vi "VariablesTCMouseDown.vi"(8 "error in (no error)":errorcluster, 10 "MouseDownIn":T3, 11 "VMUI in":refnum<class "VMUI.lvclass">) -> (0 "error out":errorcluster, 2 "MouseDownOut":T1, 3 "VMUI out":refnum<class "VMUI.lvclass">)   [LabVIEW 2013, in "VMUI.lvclass"]
uses:
  VMUI.lvclass
  <vilib>/Utility/miscctls.llb/LVPoint32TypeDef.ctl
  <vilib>/Utility/miscctls.llb/LVRowAndColumnTypeDef.ctl
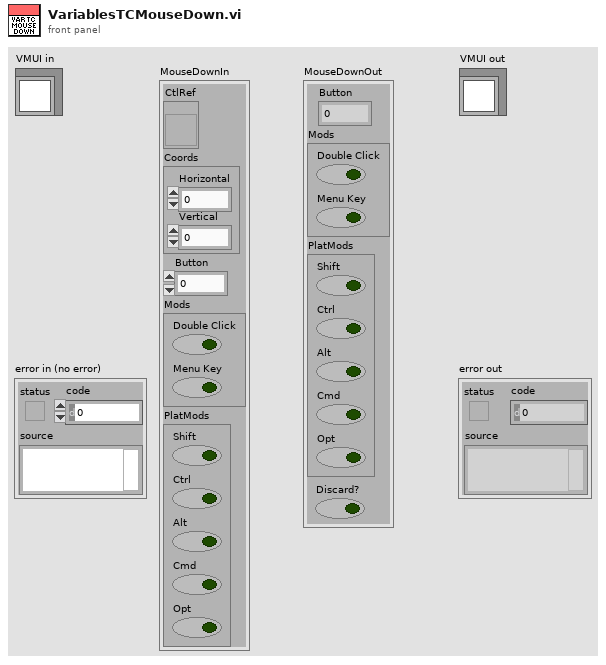
[diagram p1: front panel]
types:
  T1 = cluster{"Button":u16, "Mods":cluster{"Double Click":bool, "Menu Key":bool}, "PlatMods":cluster{"Shift":bool, "Ctrl":bool, "Alt":bool, "Cmd":bool, "Opt":bool}, "Discard?":bool}
  T2 = typedef "LVPoint32TypeDef.ctl" = cluster{"Horizontal":i32, "Vertical":i32}
  T3 = cluster{"CtlRef":refnum<vi>, "Coords":T2, "Button":u16, "Mods":cluster{"Double Click":bool, "Menu Key":bool}, "PlatMods":cluster{"Shift":bool, "Ctrl":bool, "Alt":bool, "Cmd":bool, "Opt":bool}}
  T4 = typedef "LVRowAndColumnTypeDef.ctl" = cluster{"Row":i32, "Column":i32}
  T5 = cluster{"Shift":bool, "Ctrl":bool, "Alt":bool, "Cmd":bool, "Opt":bool}
  T6 = cluster{"Button":u16, "Mods":cluster{"Double Click":bool, "Menu Key":bool}, "PlatMods":cluster{"Shift":bool, "Ctrl":bool, "Alt":bool, "Cmd":bool, "Opt":bool}, bool}
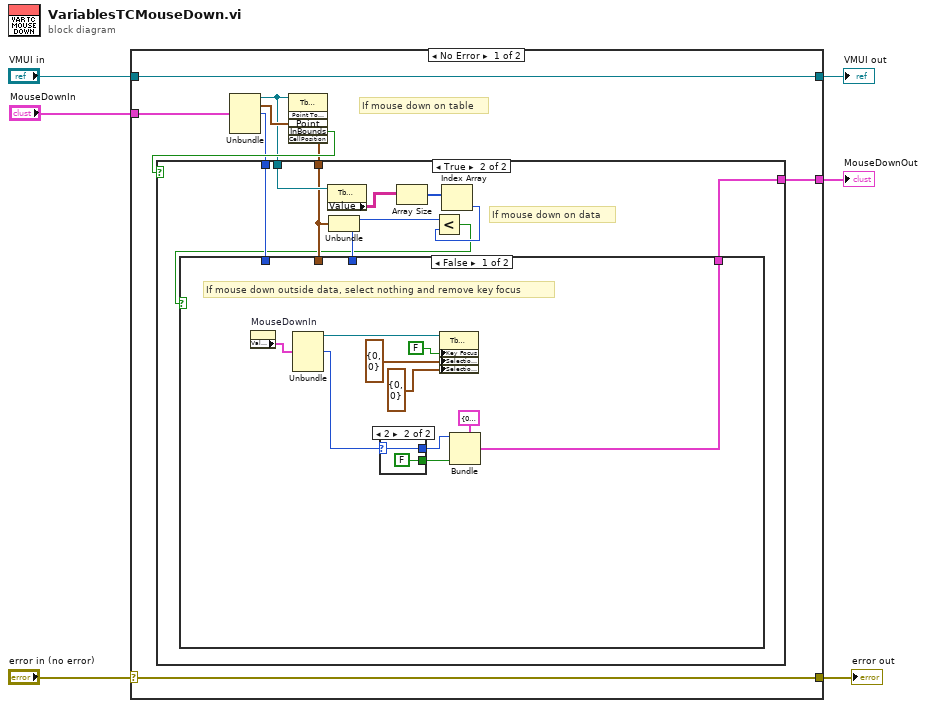
[diagram p0: block diagram]
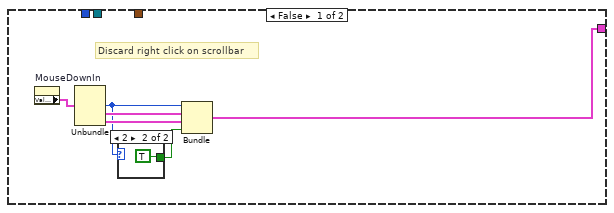
[diagram p2: hidden frame]
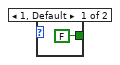
[diagram p3: hidden frame]
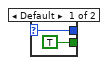
[diagram p4: hidden frame]
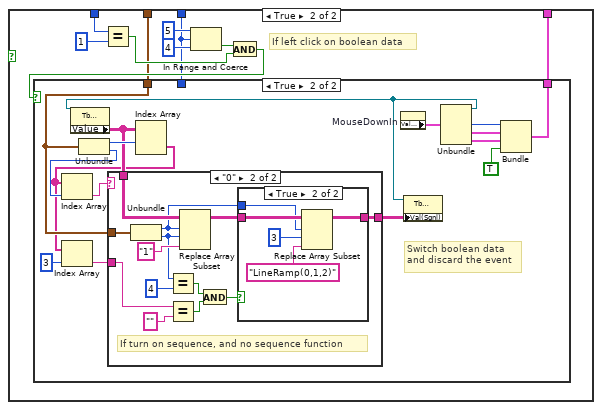
[diagram p5: hidden frame]
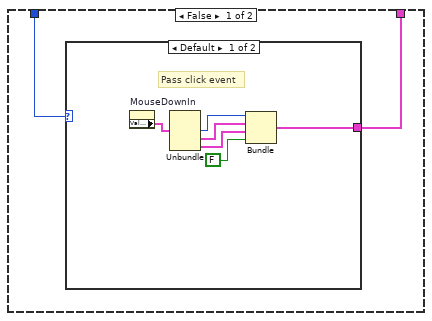
[diagram p6: hidden frame]
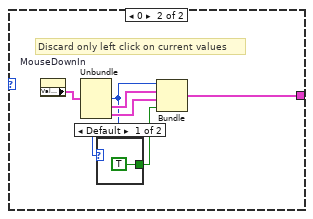
[diagram p7: hidden frame]
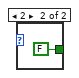
[diagram p8: hidden frame]
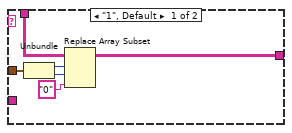
[diagram p9: hidden frame]
diagram:
  n1 = case shown="No Error" "error in (no error)" {
    selector: "error in (no error)" -> [w14 w116]
    tunnel: [w14 w116] -> w5
    tunnel: [w15 w115] -> w1
    tunnel: "VMUI in" -> [w15 w115]
    tunnel: "MouseDownIn" -> [w8 _]
    tunnel: [w7 _] -> w3
    frame No Error {
      # "If mouse down on table"
      n2 = Unbundle(w8) -> ("CtlRef"=w9:refnum<vi>, "Coords"=w13:T2, "Button"=w10:u16)  [unwired: 2 out]
      n3 = invoke class="Tbl (strict)" method="Point To Row Column"(reference=w9, "Point"=w13) -> ("InBounds"=w12:bool, "CellPosition"=w11:T4)  [unwired: 4 in, 4 out]
      n4 = case shown="True" w12 {
        tunnel: [w21 w29] -> w7
        tunnel: w11 -> [_ w26]
        tunnel: w9 -> [_ w28]
        tunnel: w10 -> [_ w27]
        frame False {
          # "Discard right click on scrollbar"
          n5 = property on="MouseDownIn" class="Clust (strict)"() -> ("Value"=w20:T3)  [unwired: 2 in, 2 out]
          n6 = Unbundle(w20) -> ("Button"=w17:u16, "Mods"=w19:cluster{"Double Click":bool, "Menu Key":bool}, "PlatMods"=w18:T5)  [unwired: 2 out]
          n7 = case shown="2" w17 {
            tunnel: [FALSE TRUE] -> w16
            frame 1, Default {
            }
            frame 2 {
            }
          }
          n8 = Bundle("Button"=w17, "Mods"=w19, "PlatMods"=w18, w16) -> (w21:T6)  [unwired: 1 in]
        }
        frame True {
          # "If mouse down on data"
          n9 = property class="Tbl (strict)"(reference=w28) -> ("Value"=w33:string[][])  [unwired: 1 in, 2 out]
          n10 = Unbundle(w26) -> ("Row"=w30:i32, "Column"=w25:i32)
          n11 = Array Size(array=w33) -> (size(s)=w32:i32[])
          n12 = Index Array(array=w32) -> (element=w31:i32)  [unwired: 1 in]
          n13 = Less?(x=w30, y=w31) -> (x < y?=w24:bool)
          n14 = case shown="False" w24 {
            tunnel: [w42 w55] -> w29
            tunnel: w25 -> [_ w48]
            tunnel: w27 -> [_ w54]
            tunnel: w26 -> [_ w49]
            frame False {
              # "If mouse down outside data, select nothing and remove key focus"
              n15 = property on="MouseDownIn" class="Clust (strict)"() -> ("Value"=w43:T3)  [unwired: 2 in, 2 out]
              n16 = Unbundle(w43) -> ("CtlRef"=w41:refnum<vi>, "Button"=w37:u16)  [unwired: 3 out]
              n17 = case shown="2" w37 {
                selector: w37 -> [w45 w46]
                tunnel: [TRUE FALSE] -> w36
                tunnel: [w45 w46] -> w35
                frame Default {
                }
                frame 2 {
                }
              }
              n18 = property class="Tbl (strict)"(reference=w41, "Key Focus"=FALSE, "Selection Size"=T4 {"Row"=0, "Column"=0}, "Selection Start"=T4 {"Row"=0, "Column"=0}) -> ()  [unwired: 1 in, 2 out]
              n19 = Bundle(cluster=T1 {"Button"=0, "Mods"={"Double Click"=FALSE, "Menu Key"=FALSE}, "PlatMods"={"Shift"=FALSE, "Ctrl"=FALSE, "Alt"=FALSE, "Cmd"=FALSE, "Opt"=FALSE}, "Discard?"=TRUE} ("MouseDownOut"), "Button"=w35, "Discard?"=w36) -> (w42:T1)  [unwired: 2 in]
            }
            frame True {
              # "If left click on boolean data"
              n20 = Equal?(x=w54, y=u16 1) -> (x = y?=w50:bool)
              n21 = In Range and Coerce(upper limit=5, x=w48, lower limit=4 ("upper limit")) -> (In Range?=w52:bool)  [unwired: 1 out]
              n22 = And(x=w52, y=w50) -> (x .and. y?=w51:bool)
              n23 = case shown="True" w51 {
                tunnel: [w59 w84] -> w55
                tunnel: w49 -> [_ w81]
                tunnel: w48 -> [w58 _]
                frame False {
                  n24 = case shown="Default" w58 {
                    tunnel: [w62 w67] -> w59
                    frame Default {
                      # "Pass click event"
                      n25 = property on="MouseDownIn" class="Clust (strict)"() -> ("Value"=w65:T3)  [unwired: 2 in, 2 out]
                      n26 = Unbundle(w65) -> ("Button"=w61:u16, "Mods"=w64:cluster{"Double Click":bool, "Menu Key":bool}, "PlatMods"=w63:T5)  [unwired: 2 out]
                      n27 = Bundle("Button"=w61, "Mods"=w64, "PlatMods"=w63, FALSE) -> (w62:T6)  [unwired: 1 in]
                    }
                    frame 0 {
                      # "Discard only left click on current values"
                      n28 = property on="MouseDownIn" class="Clust (strict)"() -> ("Value"=w70:T3)  [unwired: 2 in, 2 out]
                      n29 = Unbundle(w70) -> ("Button"=w66:u16, "Mods"=w69:cluster{"Double Click":bool, "Menu Key":bool}, "PlatMods"=w68:T5)  [unwired: 2 out]
                      n30 = case shown="Default" w66 {
                        tunnel: [TRUE FALSE] -> w71
                        frame Default {
                        }
                        frame 2 {
                        }
                      }
                      n31 = Bundle("Button"=w66, "Mods"=w69, "PlatMods"=w68, w71) -> (w67:T6)  [unwired: 1 in]
                    }
                  }
                }
                frame True {
                  # "Switch boolean data \nand discard the event"
                  n32 = Unbundle(w81) -> ("Row"=w83:i32, "Column"=w79:i32)
                  n33 = property on="MouseDownIn" class="Clust (strict)"() -> ("Value"=w88:T3)  [unwired: 2 in, 2 out]
                  n34 = Unbundle(w88) -> ("CtlRef"=w74:refnum<vi>, "Button"=w87:u16, "Mods"=w86:cluster{"Double Click":bool, "Menu Key":bool}, "PlatMods"=w85:T5)  [unwired: 1 out]
                  n35 = property class="Tbl (strict)"(reference=w74) -> ("Value"=w82:string[][])  [unwired: 1 in, 2 out]
                  n36 = Index Array(array=w82, index (row)=w83) -> (element=w77:string[])  [unwired: 1 in]
                  n37 = Index Array(array=w77, index=w79) -> (element=w78:string)
                  n38 = Index Array(array=w77, index=3) -> (element=w75:string)
                  n39 = case shown="\"0\"" w78 {
                    tunnel: w82 -> [w95 w104]
                    tunnel: w81 -> [w94 w108]
                    tunnel: [w90 w98] -> w80
                    tunnel: w75 -> [_ w103]
                    frame "1", Default {
                      n40 = Unbundle(w94) -> ("Row"=w93:i32, "Column"=w92:i32)
                      n41 = Replace Array Subset(array=w95, new element="0" ("new element/subarray"), index (row)=w93, index (col)=w92) -> (w90:string[][])
                    }
                    frame "0" {
                      # "If turn on sequence, and no sequence function"
                      n42 = Unbundle(w108) -> ("Row"=w96:i32, "Column"=w106:i32)
                      n43 = Equal?(x=w106, y=4) -> (x = y?=w101:bool)
                      n44 = Equal?(x=w103, y="") -> (x = y?=w100:bool)
                      n45 = Replace Array Subset(array=w104, new element="1" ("new element/subarray"), index (row)=w96, index (col)=w106) -> (w99:string[][])
                      n46 = And(x=w101, y=w100) -> (x .and. y?=w97:bool)
                      n47 = case shown="True" w97 {
                        tunnel: w99 -> [w109 w114]
                        tunnel: [w109 w113] -> w98
                        tunnel: w96 -> [_ w112]
                        frame False {
                        }
                        frame True {
                          n48 = Replace Array Subset(array=w114, new element="LineRamp(0,1,2)", index (row)=w112, index (col)=3 ("disabled index (col)")) -> (w113:string[][])
                        }
                      }
                    }
                  }
                  n49 = property class="Tbl (strict)"(reference=w74, "Val(Sgnl)"=w80) -> ()  [unwired: 1 in, 2 out]
                  n50 = Bundle("Button"=w87, "Mods"=w86, "PlatMods"=w85, TRUE) -> (w84:T6)  [unwired: 1 in]
                }
              }
            }
          }
        }
      }
    }
    frame Error {
    }
  }
  "error out" <- w5
  "VMUI out" <- w1
  "MouseDownOut" <- w3
